vi "CSC_SetEndEff.vi"(8 "error in (no error)":errorcluster, 10 "Point":T1={"Coord4"=[0.0, 0.0, 0.0, 1.0], "ID"=0}, 11 "CableSerialChain in":refnum<class "CableSerialChain.lvclass">) -> (0 "error out":errorcluster, 3 "CableSerialChain out":refnum<class "CableSerialChain.lvclass">)   [LabVIEW 2015, in "CableSerialChain.lvclass"]
uses:
  CableSerialChain.lvclass
  Body/PointOnBody.ctl
  CableSerialChain.lvclass/CableSerialChain.ctl
  Body/Bodies.lvclass
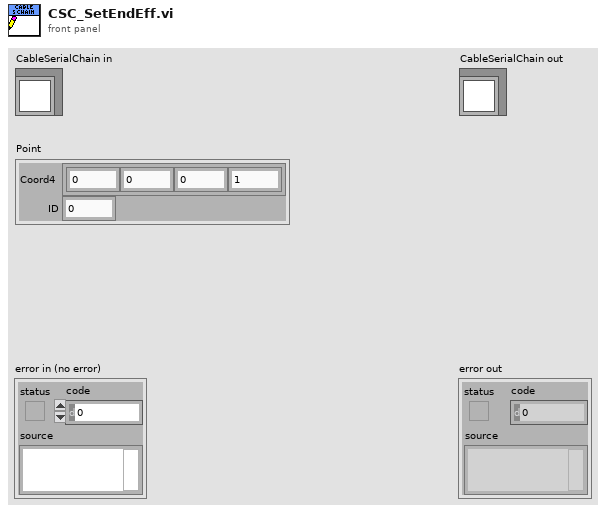
[diagram p1: front panel]
types:
  T1 = typedef "Bodies.lvclass/PointOnBody.ctl" = cluster{"Coord4":dbl[], "ID":i32}
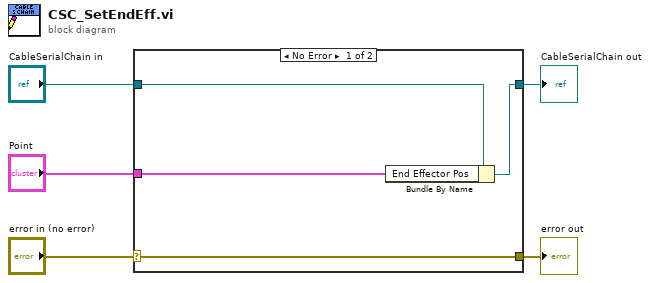
[diagram p0: block diagram]
diagram:
  n1 = case shown="No Error" "error in (no error)" {
    selector: "error in (no error)" -> [w9 w10]
    tunnel: [w9 w10] -> w4
    tunnel: [w7 w11] -> w2
    tunnel: "CableSerialChain in" -> [w8 w11]
    tunnel: "Point" -> [w6 _]
    frame No Error {
      n2 = Bundle By Name(cluster=w8, "End Effector Pos"=w6) -> (w7:refnum<class "CableSerialChain.lvclass">)
    }
    frame Error {
    }
  }
  "error out" <- w4
  "CableSerialChain out" <- w2
